vi "QueryServer_Start.vi"(7 "error in (no error)":errorcluster, 8 "Server Key File (.key)":path, 9 "Server Certificate File (.crt)":path, 10 "Server Address":string) -> (0 "error out":errorcluster, 2 "Event Registration Refnum":refnum<event-registration>, 3 "Server Information":T2)   [LabVIEW 2019, in "labview-grpc-query-server.lvlib"]
uses:
  labview-grpc-query-server.lvlib
  QueryServer_InvokeEventData.ctl
  QueryServer_gRPCid.ctl
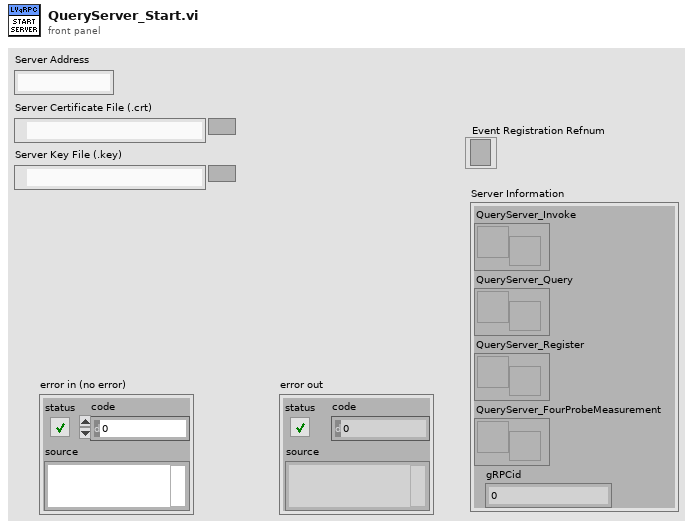
[diagram p1: front panel]
types:
  T1 = typedef "labview-grpc-query-server.lvlib/QueryServer_gRPCid.ctl" = u64
  T2 = cluster{"QueryServer_Invoke":refnum<user-event>, "QueryServer_Query":refnum<user-event>, "QueryServer_Register":refnum<user-event>, "QueryServer_FourProbeMeasurement":refnum<user-event>, "gRPCid":T1}
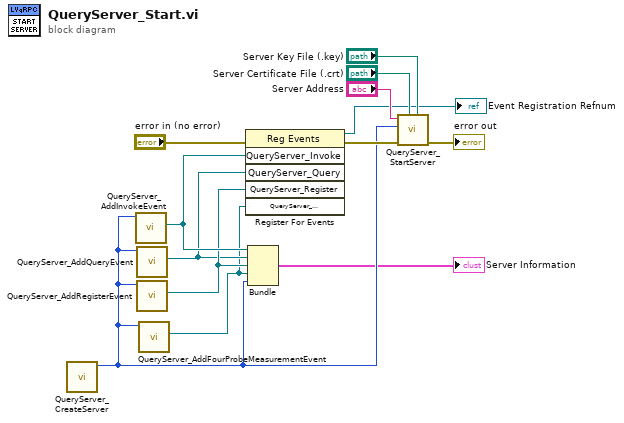
[diagram p0: block diagram]
diagram:
  n1 = call "QueryServer_CreateServer.vi"() -> ("gRPCid"=w4:T1)  [unwired: 11 in]
  n2 = call "QueryServer_AddInvokeEvent.vi"("gRPCid in"=w4) -> ("QueryServer_Invoke"=w9:refnum<user-event>)  [unwired: 9 in, 1 out]
  n3 = call "QueryServer_AddQueryEvent.vi"("gRPCid in"=w4) -> ("QueryServer_Query"=w7:refnum<user-event>)  [unwired: 9 in, 1 out]
  n4 = call "QueryServer_AddRegisterEvent.vi"("gRPCid in"=w4) -> ("QueryServer_Register"=w8:refnum<user-event>)  [unwired: 9 in, 1 out]
  n5 = call "QueryServer_AddFourProbeMeasurementEvent.vi"("gRPCid in"=w4) -> ("QueryServer_FourProbeMeasurement"=w3:refnum<user-event>)  [unwired: 9 in, 1 out]
  n6 = register-events(error in="error in (no error)", w9, w7, w8, w3) -> (reference out=→"Event Registration Refnum":refnum<event-registration>, error out=w12:errorcluster)  [unwired: 1 in]
  n7 = Bundle("QueryServer_Invoke"=w9, "QueryServer_Query"=w7, "QueryServer_Register"=w8, "QueryServer_FourProbeMeasurement"=w3, "gRPCid"=w4) -> (→"Server Information":T2)  [unwired: 1 in]
  n8 = call "QueryServer_StartServer.vi"("Server Key File (.key)"="Server Key File (.key)", "Server Certificate File (.crt)"="Server Certificate File (.crt)", "error in (no error)"=w12, "gRPCid"=w4, "Server Address"="Server Address") -> ("error out"=→"error out":errorcluster)  [unwired: 6 in]
